vi "Next Clock.vi"(8 "error in (no error)":errorcluster, 11 "Clock Generator in":refnum<class "IO.lvclass">) -> (0 "error out":errorcluster, 2 "Current State":bool, 3 "Clock Generator out":refnum<class "IO.lvclass">)   [LabVIEW 2021, in "IO.lvclass"]
uses:
  IO/IO.lvclass
  IO/IO.lvclass/IO.ctl
  <vilib>/DAQmx/write.llb/DAQmx Write (Digital Bool 1Line 1Point).vi
  <vilib>/DAQmx/miscellaneous.llb/DAQmx Fill In Error Info.vi
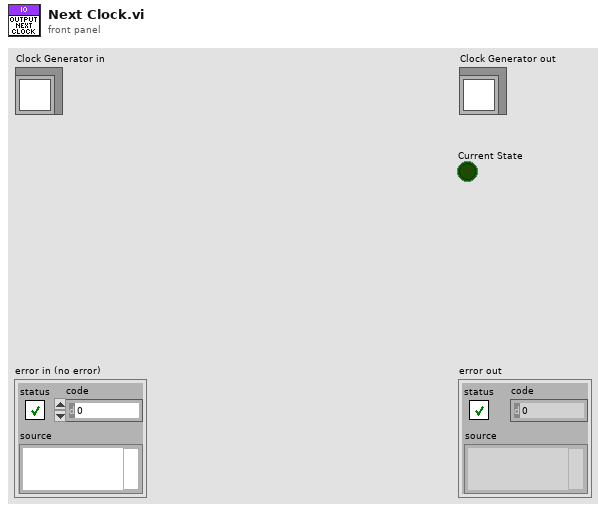
[diagram p1: front panel]
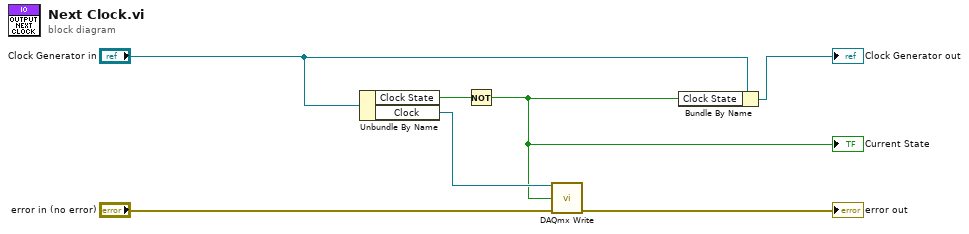
[diagram p0: block diagram]
diagram:
  n1 = Unbundle By Name("Clock Generator in") -> ("Clock State"=w5:bool, "Clock"=w2:refnum<k21>)
  n2 = Not(x=w5) -> (.not. x?=w1:bool)
  "Current State" <- w1
  n3 = call-poly <vilib>:"DAQmx Write.vi"("task/channels in"=w2, "data"=w1, "error in"="error in (no error)") -> ("error out"=→"error out":errorcluster)  [unwired: 10 in, 2 out]
  n4 = Bundle By Name(cluster="Clock Generator in", "Clock State"=w1) -> (→"Clock Generator out":refnum<class "IO.lvclass">)
